vi "BCD to Decimal.vi"(11 "word raw data - bcd":u16) -> (3 "decimal data out":u32)   [LabVIEW 2020, in "dt_encodeDecode.lvlib"]
uses:
  dt_encodeDecode.lvlib
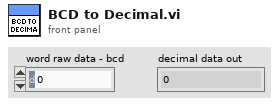
[diagram p1: front panel]
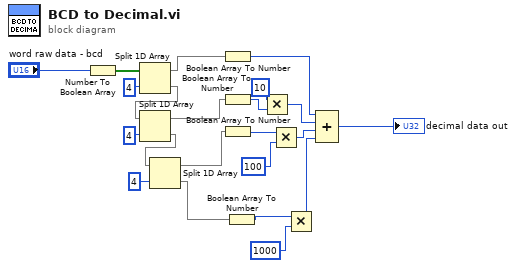
[diagram p0: block diagram]
diagram:
  n1 = Number To Boolean Array(number="word raw data - bcd") -> (Boolean array=w8:bool[])
  n2 = Split 1D Array(array=w8, index=4) -> (first subarray=w16:bool[], second subarray=w13:bool[])
  n3 = Split 1D Array(array=w13, index=4) -> (first subarray=w17:bool[], second subarray=w7:bool[])
  n4 = Split 1D Array(array=w7, index=4) -> (first subarray=w6:bool[], second subarray=w4:bool[])
  n5 = Boolean Array To Number(Boolean array=w16) -> (number=w18:u32)
  n6 = Boolean Array To Number(Boolean array=w17) -> (number=w11:u32)
  n7 = Boolean Array To Number(Boolean array=w6) -> (number=w19:u32)
  n8 = Boolean Array To Number(Boolean array=w4) -> (number=w2:u32)
  n9 = Multiply(x=u32 10, y=w11) -> (x*y=w10:u32)
  n10 = Multiply(x=w19, y=u32 100 ("x")) -> (x*y=w21:u32)
  n11 = Multiply(x=w2, y=u32 1000 ("x")) -> (x*y=w1:u32)
  n12 = Compound Arithmetic op=ADD(w18, w10, w21, w1) -> (→"decimal data out":u32)
